vi "Read I16.vi"(8 "error in":errorcluster, 10 "register name":string, 11 "session in":u32) -> (0 "error out":errorcluster, 2 "value out":i16, 3 "session out":u32)   [LabVIEW 2018, in "Scalar IO Operations.lvlib"]
uses:
  Scalar IO Operations.lvlib
  NiFpga.dll
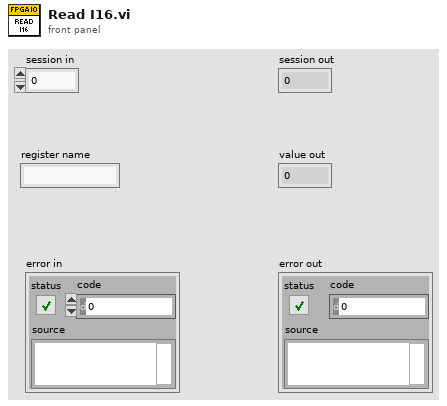
[diagram p1: front panel]
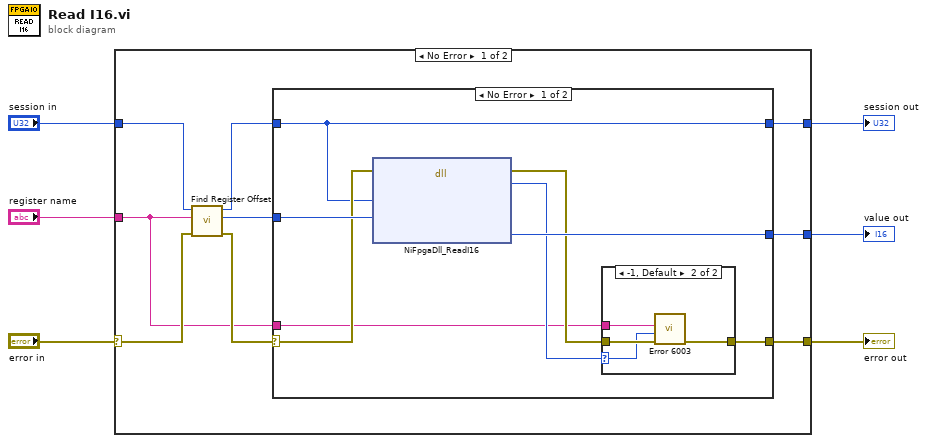
[diagram p0: block diagram]
diagram:
  n1 = case shown="No Error" "error in" {
    selector: "error in" -> [w8 w31]
    tunnel: [w15 w31] -> w6
    tunnel: [w14 _] -> w5
    tunnel: [w13 w32] -> w4
    tunnel: "session in" -> [w11 w32]
    tunnel: "register name" -> [w7 _]
    frame No Error {
      n2 = call "Find Register Offset.vi"("error in (no error)"=w8, "register name"=w7, "session in"=w11) -> ("error out"=w12:errorcluster, "resource offset"=w9:u32, "session out"=w10:u32)  [unwired: 6 in]
      n3 = case shown="No Error" w12 {
        selector: w12 -> [w21 w30]
        tunnel: w10 -> [w20 w29]
        tunnel: [w19 w30] -> w15
        tunnel: [w23 _] -> w14
        tunnel: w9 -> [w22 _]
        tunnel: [w20 w29] -> w13
        tunnel: w7 -> [w16 _]
        frame No Error {
          n4 = dll-call lib="NiFpga.*" fn="NiFpgaDll_ReadI16"(error in=w21, "session"=w20, "offset"=w22) -> (error out=w18:errorcluster, "status"=w17:i32, "value"=w23:i16)  [unwired: 5 in, 1 out]
          n5 = case shown="-1, Default" w17 {
            selector: w17 -> [_ w25]
            tunnel: w18 -> [w24 w28]
            tunnel: [w24 w27] -> w19
            tunnel: w16 -> [_ w26]
            frame 0 {
            }
            frame -1, Default {
              n6 = call "Error 6003.vi"("error in (no error)"=w28, "rio status code"=w25, "register name"=w26) -> ("error out"=w27:errorcluster)  [unwired: 8 in]
            }
          }
        }
        frame Error {
        }
      }
    }
    frame Error {
    }
  }
  "error out" <- w6
  "session out" <- w4
  "value out" <- w5
